vi "GetTemplatePath.vi"(0 "ClassWriterIn":refnum<class "ClassWriter.lvclass">, 1 "ClassTemplateSubDirectory":string, 5 "error in (no error)":errorcluster) -> (14 "ClassWriterOut":refnum<class "ClassWriter.lvclass">, 15 "FolderPathOut":path, 17 "MethodTemplatePathOut":path, 18 "TemplateSettings":T1, 19 "error out":errorcluster)   [LabVIEW 2012, in "ClassWriter.lvclass"]
uses:
  <resource>/Framework/Providers/Open_GDS/ClassProviders/Provider_BaseClassInterface/ClassWriter_class/ClassWriter.lvclass
  <resource>/Framework/Providers/Open_GDS/ClassProviders/Provider_BaseClassInterface/ClassWriter_class/TemplateSettings.ctl
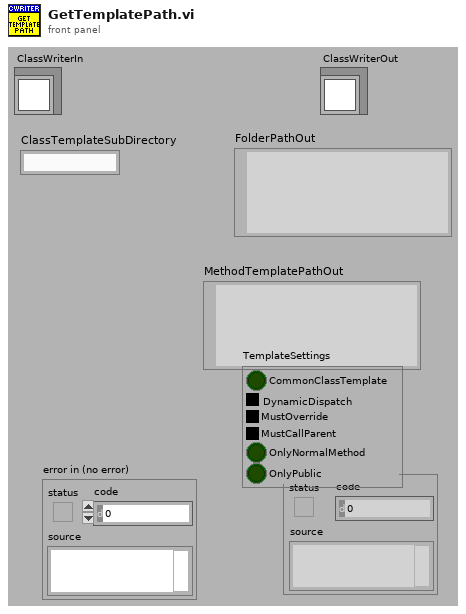
[diagram p1: front panel]
types:
  T1 = typedef "ClassWriter.lvclass/TemplateSettings.ctl" = cluster{"CommonClassTemplate":bool, "DynamicDispatch":enum8{"False", "True", "Mixed"}, "MustOverride":enum8{"False", "True", "Mixed"}, "MustCallParent":enum8{"False", "True", "Mixed"}, "OnlyNormalMethod":bool, "OnlyPublic":bool}
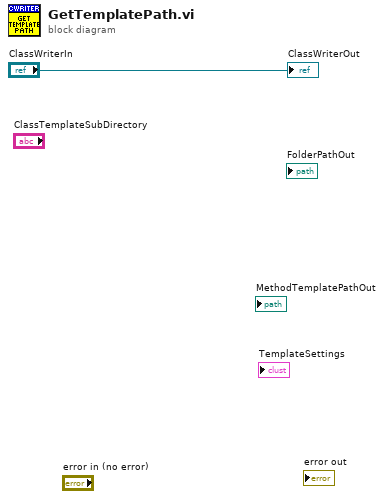
[diagram p0: block diagram]
diagram:
  "ClassWriterOut" <- "ClassWriterIn"
